vi "Frameremap.vi"(0 "Frame Origin (m)":cluster{"Xc":sgl, "Yc":sgl} {"Yc" format="%.2p"; "Xc" format="%.2p"}, 1 "Frame Size (m)":cluster{"Width":sgl, "Height":sgl} {"Height" format="%.2p"; "Width" format="%.2p"}) -> (7 "Frame Properties (Remapped)":T1)   [LabVIEW 2017]
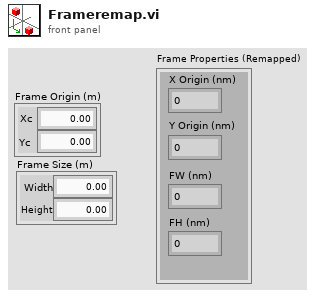
[diagram p1: front panel]
types:
  T1 = cluster{"X Origin (nm)":dbl, "Y Origin (nm)":dbl, "FW (nm)":dbl, "FH (nm)":dbl}
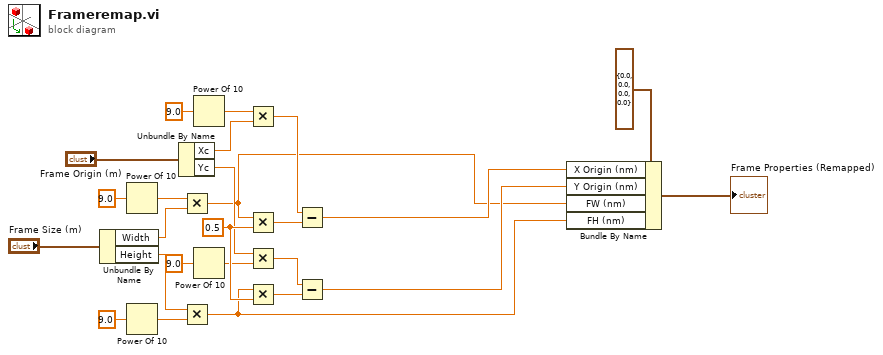
[diagram p0: block diagram]
diagram:
  w25 = 0.5 ("y")
  n1 = Unbundle By Name("Frame Size (m)") -> ("Width"=w19:sgl, "Height"=w16:sgl)
  n2 = Power Of 10(x=9.0) -> (10^x=w20:dbl)
  n3 = Power Of 10(x=9.0) -> (10^x=w18:dbl)
  n4 = Unbundle By Name("Frame Origin (m)") -> ("Xc"=w10:sgl, "Yc"=w9:sgl)
  n5 = Multiply(x=w20, y=w19) -> (x*y=w4:dbl)
  n6 = Multiply(x=w16, y=w18) -> (x*y=w3:dbl)
  n7 = Power Of 10(x=9.0) -> (10^x=w13:dbl)
  n8 = Power Of 10(x=9.0) -> (10^x=w12:dbl)
  n9 = Multiply(x=w13, y=w10) -> (x*y=w8:dbl)
  n10 = Multiply(x=w4, y=w25) -> (x*y=w24:dbl)
  n11 = Multiply(x=w9, y=w12) -> (x*y=w7:dbl)
  n12 = Multiply(x=w3, y=w25) -> (x*y=w23:dbl)
  n13 = Subtract(x=w8, y=w24) -> (x-y=w6:dbl)
  n14 = Subtract(x=w7, y=w23) -> (x-y=w5:dbl)
  n15 = Bundle By Name(cluster=T1 {"X Origin (nm)"=0.0, "Y Origin (nm)"=0.0, "FW (nm)"=0.0, "FH (nm)"=0.0} ("Cluster"), "X Origin (nm)"=w6, "Y Origin (nm)"=w5, "FW (nm)"=w4, "FH (nm)"=w3) -> (→"Frame Properties (Remapped)":T1)
